vi "BX.Init__LCR.vi"(3 "Container State":T10, 4 "Previous State":variant, 5 "Previous Version":T9) -> (2 "Current State":T1={"Orientation"=0, "ActivePicture"={"image type"=0, "image depth"=0, "image"=[], "mask"=[], "colors"=[], "Rectangle"={"left"=0, "top"=0, "right"=0, "bottom"=0}}, "Pictures"={"Normal"={"image type"=0, "image depth"=0, "image"=[], "mask"=[], "colors"=[], "Rectangle"={"left"=0, "top"=0, "right"=0, "bottom"=0}}, "Hilite"={"image type"=0, "image depth"=0, "image"=[], "mask"=[], "colors"=[], "Rectangle"={"left"=0, "top"=0, "right"=0, "bottom"=0}}}, "Text"={"String"="", "Font"={"Font Name:"="", "Size"=0, "Strikeout?"=FALSE, "Italic?"=FALSE, "Underline?"=FALSE, "Outline?"=FALSE, "Shadow?"=FALSE, "Bold?"=FALSE}, "TextColor"=0}, "RunTimeSettings"={"Highlight"=FALSE, "ShowButton"=TRUE, "Behaviour"=enum."Switch when pressed", "React if disabled"=FALSE, "Nudge Button"=TRUE, "ShowButton on Hover"=FALSE, "Button Type"=enum."System"}, "Messages"=[], "Status"=0, "XControl Label"="", "Boolean Value"=FALSE} {"Status" format="%.0x"})   [LabVIEW 2011, in "BooleanXControl__LCR.xctl"]
doc: "Loads data from the owning VI into the XControl"
uses:
  BooleanXControl__LCR.xctl
  BX.State__LCR.ctl
  Controls/BX.Orientation__LCR.ctl
  <vilib>/picture/picture.llb/imagedata.ctl
  Controls/BX.RTSettings__LCR.ctl
  Controls/BX.Behaviour__LCR.ctl
  Controls/BX.ButtonType__LCR.ctl
  Controls/BX.Message__LCR.ctl
  Controls/BX.Commands__LCR.ctl
  <vilib>/_xctls/Container State.ctl
  <vilib>/_xctls/Version.ctl
  <vilib>/_xctls/XControlSupport.lvlib
panel:
  in  "Default Indicator State":T1={"Orientation"=0, "ActivePicture"={"image type"=0, "image depth"=0, "image"=[], "mask"=[], "colors"=[], "Rectangle"={"left"=0, "top"=0, "right"=0, "bottom"=0}}, "Pictures"={"Normal"={"image type"=0, "image depth"=0, "image"=[], "mask"=[], "colors"=[], "Rectangle"={"left"=0, "top"=0, "right"=0, "bottom"=0}}, "Hilite"={"image type"=0, "image depth"=0, "image"=[], "mask"=[], "colors"=[], "Rectangle"={"left"=0, "top"=0, "right"=0, "bottom"=0}}}, "Text"={"String"="", "Font"={"Font Name:"="", "Size"=10, "Strikeout?"=FALSE, "Italic?"=FALSE, "Underline?"=FALSE, "Outline?"=FALSE, "Shadow?"=FALSE, "Bold?"=FALSE}, "TextColor"=0}, "RunTimeSettings"={"Highlight"=TRUE, "ShowButton"=TRUE, "Behaviour"=enum."Switch when pressed", "React if disabled"=FALSE, "Nudge Button"=TRUE, "ShowButton on Hover"=FALSE, "Button Type"=enum."System"}, "Messages"=[], "Status"=0, "XControl Label"="", "Boolean Value"=FALSE} {"Status" format="%.0x"}
  in  "Default Control State":T1={"Orientation"=0, "ActivePicture"={"image type"=0, "image depth"=0, "image"=[], "mask"=[], "colors"=[], "Rectangle"={"left"=0, "top"=0, "right"=0, "bottom"=0}}, "Pictures"={"Normal"={"image type"=0, "image depth"=0, "image"=[], "mask"=[], "colors"=[], "Rectangle"={"left"=0, "top"=0, "right"=0, "bottom"=0}}, "Hilite"={"image type"=0, "image depth"=0, "image"=[], "mask"=[], "colors"=[], "Rectangle"={"left"=0, "top"=0, "right"=0, "bottom"=0}}}, "Text"={"String"="", "Font"={"Font Name:"="", "Size"=10, "Strikeout?"=FALSE, "Italic?"=FALSE, "Underline?"=FALSE, "Outline?"=FALSE, "Shadow?"=FALSE, "Bold?"=FALSE}, "TextColor"=0}, "RunTimeSettings"={"Highlight"=TRUE, "ShowButton"=TRUE, "Behaviour"=enum."Switch when pressed", "React if disabled"=FALSE, "Nudge Button"=TRUE, "ShowButton on Hover"=FALSE, "Button Type"=enum."System"}, "Messages"=[], "Status"=0, "XControl Label"="", "Boolean Value"=FALSE} {"Status" format="%.0x"}
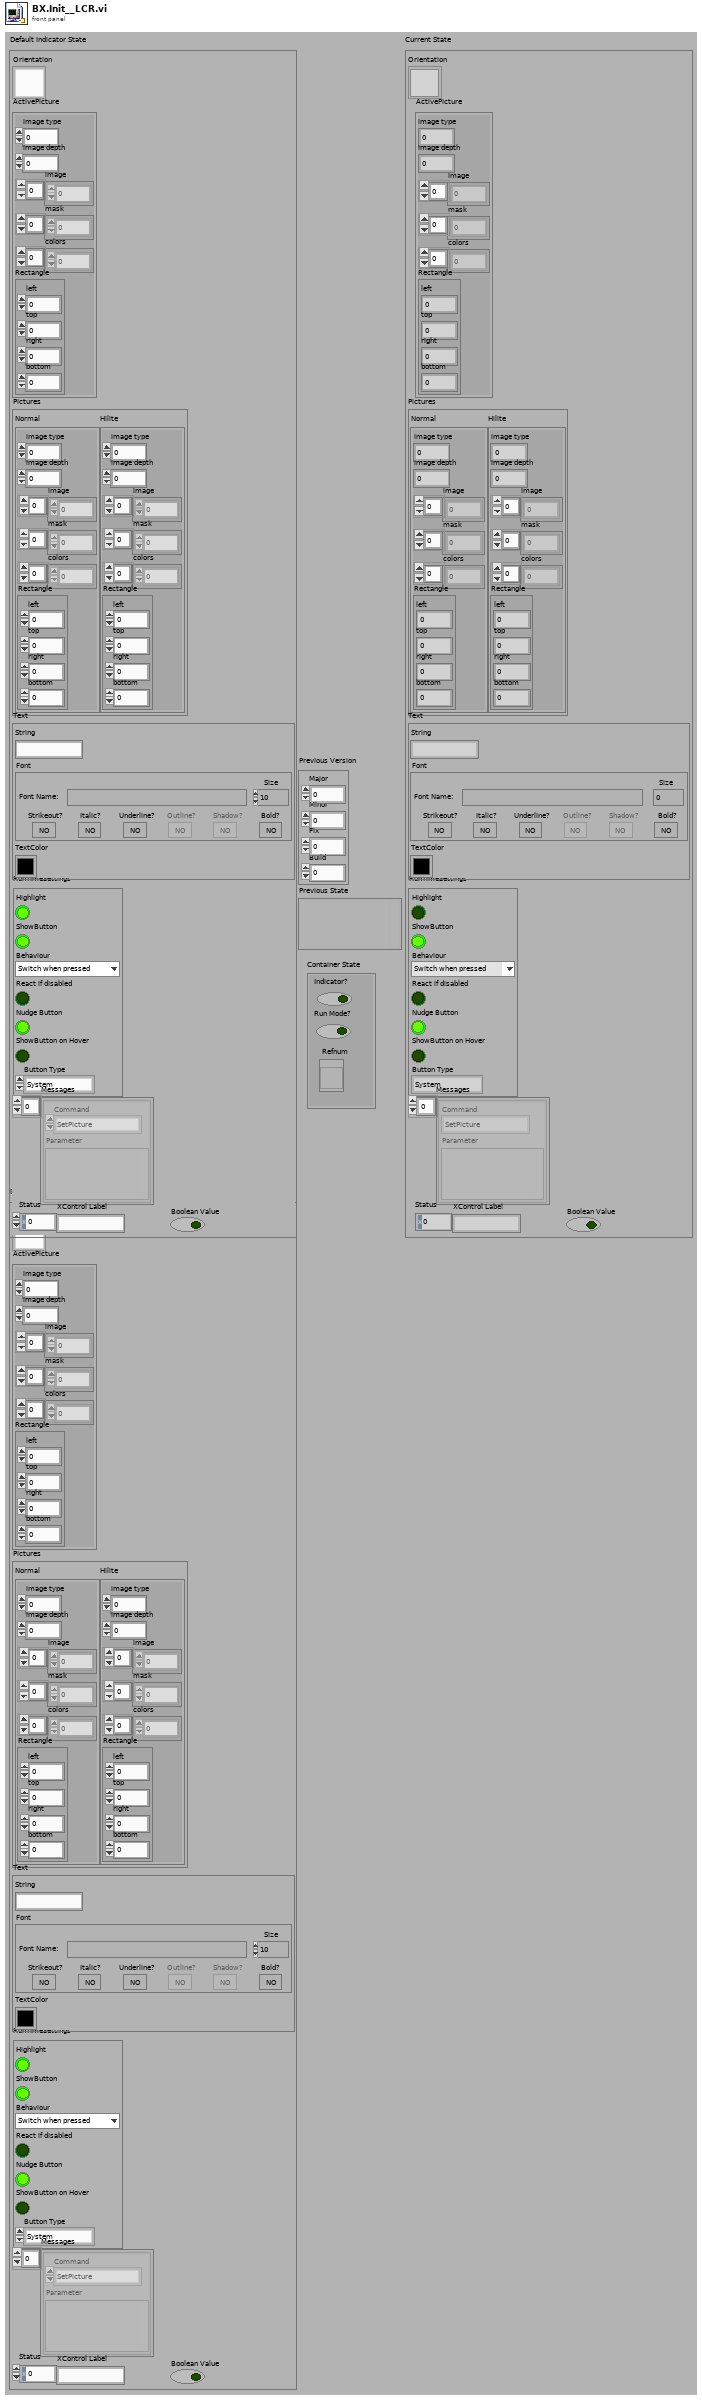
[diagram p1: front panel]
types:
  T1 = typedef "BooleanXControl__LCR.xctl/BX.State__LCR.ctl" = cluster{"Orientation":T2, "ActivePicture":T3, "Pictures":cluster{"Normal":T3, "Hilite":T3}, "Text":cluster{"String":string, "Font":cluster{"Font Name:":string, "Size":i16, "Strikeout?":bool, "Italic?":bool, "Underline?":bool, "Outline?":bool, "Shadow?":bool, "Bold?":bool}, "TextColor":u32}, "RunTimeSettings":T4, "Messages":T7[], "Status":u16, "XControl Label":string, "Boolean Value":bool}
  T2 = typedef "BooleanXControl__LCR.xctl/BX.Orientation__LCR.ctl" = u8
  T3 = typedef "imagedata.ctl" = cluster{"image type":i32, "image depth":i32, "image":u8[], "mask":u8[], "colors":u32[], "Rectangle":cluster{"left":i16, "top":i16, "right":i16, "bottom":i16}}
  T4 = typedef "BooleanXControl__LCR.xctl/BX.RTSettings__LCR.ctl" = cluster{"Highlight":bool, "ShowButton":bool, "Behaviour":T5, "React if disabled":bool, "Nudge Button":bool, "ShowButton on Hover":bool, "Button Type":T6}
  T5 = typedef "BooleanXControl__LCR.xctl/BX.Behaviour__LCR.ctl" = enum16{"Switch when pressed", "Switch when released", "Switch until released"}
  T6 = typedef "BooleanXControl__LCR.xctl/BX.ButtonType__LCR.ctl" = enum16{"System", "Modern", "Classic", "Decoration"}
  T7 = typedef "BooleanXControl__LCR.xctl/BX.Message__LCR.ctl" = cluster{"Command":T8, "Parameter":variant}
  T8 = typedef "BooleanXControl__LCR.xctl/BX.Commands__LCR.ctl" = enum16{"None", "SetPicture", "SetFont", "SetText", "SetOrientation", "Redraw", "SetTextColor", "SetRTSettings", "MultipleUpdate", "RT.Button", "RT.Hilite", "RT.Behaviour", "RT.Disabled", "ShowGUI", "RT.Nudge", "RT.Hover", "RT.ButtonType"}
  T9 = typedef "XControlSupport.lvlib/Version.ctl" = cluster{"Major":u16, "Minor":u16, "Fix":u16, "Build":u16}
  T10 = typedef "XControlSupport.lvlib/Container State.ctl" = cluster{"Indicator?":bool, "Run Mode?":bool, " Refnum":refnum<vi>}
  T11 = cluster{"Orientation":u8, "ActivePicture":cluster{"image type":i32, "image depth":i32, "image":u8[], "mask":u8[], "colors":u32[], "Rectangle":cluster{"left":i16, "top":i16, "right":i16, "bottom":i16}}, "Pictures":cluster{"Normal":cluster{"image type":i32, "image depth":i32, "image":u8[], "mask":u8[], "colors":u32[], "Rectangle":cluster{"left":i16, "top":i16, "right":i16, "bottom":i16}}, "Hilite":cluster{"image type":i32, "image depth":i32, "image":u8[], "mask":u8[], "colors":u32[], "Rectangle":cluster{"left":i16, "top":i16, "right":i16, "bottom":i16}}}, "Text":cluster{"String":string, "Font":cluster{"Font Name:":string, "Size":i16, "Strikeout?":bool, "Italic?":bool, "Underline?":bool, "Outline?":bool, "Shadow?":bool, "Bold?":bool}, "TextColor":u32}, "RunTimeSettings":cluster{"Highlight":bool, "ShowButton":bool, "Behaviour":T5, "React if disabled":bool}, "Messages":cluster{"Command":enum16{"None", "SetPicture", "SetFont", "SetText", "SetOrientation", "Redraw", "SetTextColor", "SetRTSettings", "MultipleUpdate", "RT.Button", "RT.Hilite", "RT.Behaviour", "RT.Disabled", "ShowGUI"}, "Parameter":variant}[], "Status":u16, "XControl Label":string}
  T12 = cluster{"Orientation":u8, "ActivePicture":cluster{"image type":i32, "image depth":i32, "image":u8[], "mask":u8[], "colors":u32[], "Rectangle":cluster{"left":i16, "top":i16, "right":i16, "bottom":i16}}, "Pictures":cluster{"Normal":cluster{"image type":i32, "image depth":i32, "image":u8[], "mask":u8[], "colors":u32[], "Rectangle":cluster{"left":i16, "top":i16, "right":i16, "bottom":i16}}, "Hilite":cluster{"image type":i32, "image depth":i32, "image":u8[], "mask":u8[], "colors":u32[], "Rectangle":cluster{"left":i16, "top":i16, "right":i16, "bottom":i16}}}, "Text":cluster{"String":string, "Font":cluster{"Font Name:":string, "Size":i16, "Strikeout?":bool, "Italic?":bool, "Underline?":bool, "Outline?":bool, "Shadow?":bool, "Bold?":bool}, "TextColor":u32}, "RunTimeSettings":cluster{"Highlight":bool, "ShowButton":bool, "Behaviour":enum16{"Switch when pressed", "Switch when released", "Switch until released"}, "React if disabled":bool}, "Messages":cluster{"Command":T8, "Parameter":variant}, "Status":u16, "XControl Label":string, "Events (DO NOT DESTROY)":cluster{"user event":refnum<user-event>, "Event Registration Refnum":refnum<event-registration>}}
  T13 = cluster{"Orientation":u8, "ActivePicture":cluster{"image type":i32, "image depth":i32, "image":u8[], "mask":u8[], "colors":u32[], "Rectangle":cluster{"left":i16, "top":i16, "right":i16, "bottom":i16}}, "Pictures":cluster{"Normal":cluster{"image type":i32, "image depth":i32, "image":u8[], "mask":u8[], "colors":u32[], "Rectangle":cluster{"left":i16, "top":i16, "right":i16, "bottom":i16}}, "Hilite":cluster{"image type":i32, "image depth":i32, "image":u8[], "mask":u8[], "colors":u32[], "Rectangle":cluster{"left":i16, "top":i16, "right":i16, "bottom":i16}}}, "Text":cluster{"String":string, "Font":cluster{"Font Name:":string, "Size":i16, "Strikeout?":bool, "Italic?":bool, "Underline?":bool, "Outline?":bool, "Shadow?":bool, "Bold?":bool}, "TextColor":u32}, "RunTimeSettings":cluster{"Highlight":bool, "ShowButton":bool, "Behaviour":enum16{"Switch when pressed", "Switch when released", "Switch until released"}, "React if disabled":bool}, "Messages":cluster{"Command":enum16{"None", "SetPicture", "SetFont", "SetText", "SetOrientation", "Redraw", "SetTextColor", "SetRTSettings", "MultipleUpdate", "RT.Button", "RT.Hilite", "RT.Behaviour", "RT.Disabled", "ShowGUI"}, "Parameter":variant}, "Status":u16}
  T14 = cluster{"Orientation":u8, "ActivePicture":cluster{"image type":i32, "image depth":i32, "image":u8[], "mask":u8[], "colors":u32[], "Rectangle":cluster{"left":i16, "top":i16, "right":i16, "bottom":i16}}, "Pictures":cluster{"Normal":cluster{"image type":i32, "image depth":i32, "image":u8[], "mask":u8[], "colors":u32[], "Rectangle":cluster{"left":i16, "top":i16, "right":i16, "bottom":i16}}, "Hilite":cluster{"image type":i32, "image depth":i32, "image":u8[], "mask":u8[], "colors":u32[], "Rectangle":cluster{"left":i16, "top":i16, "right":i16, "bottom":i16}}}, "Text":cluster{"String":string, "Font":cluster{"Font Name:":string, "Size":i16, "Strikeout?":bool, "Italic?":bool, "Underline?":bool, "Outline?":bool, "Shadow?":bool, "Bold?":bool}, "TextColor":u32}, "RunTimeSettings":cluster{"Highlight":bool, "ShowButton":bool, "Behaviour":enum16{"Switch when pressed", "Switch when released", "Switch until released"}, "React if disabled":bool}, "Messages":cluster{"Command":enum16{"None", "SetPicture", "SetFont", "SetText", "SetOrientation", "Redraw", "SetTextColor", "SetRTSettings", "MultipleUpdate", "RT.Button", "RT.Hilite", "RT.Behaviour", "RT.Disabled", "ShowGUI"}, "Parameter":variant}, "Spacing":u8}
  T15 = cluster{"image type":i32, "image depth":i32, "image":u8[], "mask":u8[], "colors":u32[], "Rectangle":cluster{"left":i16, "top":i16, "right":i16, "bottom":i16}}
  T16 = cluster{"Normal":cluster{"image type":i32, "image depth":i32, "image":u8[], "mask":u8[], "colors":u32[], "Rectangle":cluster{"left":i16, "top":i16, "right":i16, "bottom":i16}}, "Hilite":cluster{"image type":i32, "image depth":i32, "image":u8[], "mask":u8[], "colors":u32[], "Rectangle":cluster{"left":i16, "top":i16, "right":i16, "bottom":i16}}}
  T17 = cluster{"String":string, "Font":cluster{"Font Name:":string, "Size":i16, "Strikeout?":bool, "Italic?":bool, "Underline?":bool, "Outline?":bool, "Shadow?":bool, "Bold?":bool}, "TextColor":u32}
  T18 = cluster{"Highlight":bool, "ShowButton":bool, "Behaviour":enum16{"Switch when pressed", "Switch when released", "Switch until released"}, "React if disabled":bool}
  T19 = cluster{"Command":enum16{"None", "SetPicture", "SetFont", "SetText", "SetOrientation", "Redraw", "SetTextColor", "SetRTSettings", "MultipleUpdate", "RT.Button", "RT.Hilite", "RT.Behaviour", "RT.Disabled", "ShowGUI"}, "Parameter":variant}
  T20 = enum16{"Switch when pressed", "Switch when released", "Switch until released"}
  T21 = cluster{"Command":enum16{"None", "SetPicture", "SetFont", "SetText", "SetOrientation", "Redraw", "SetTextColor", "SetRTSettings", "MultipleUpdate", "RT.Button", "RT.Hilite", "RT.Behaviour", "RT.Disabled", "ShowGUI"}, "Parameter":variant}[]
  T22 = cluster{"Highlight":bool, "ShowButton":bool, "Behaviour":enum16{"Switch when pressed", "Switch when released", "Switch until released"}, "React if disabled":bool, bool, bool, "Button Type":T6}
  T23 = cluster{"Highlight":bool, "ShowButton":bool, "Behaviour":T5, "React if disabled":bool}
  T24 = cluster{"Highlight":bool, "ShowButton":bool, "Behaviour":T5, "React if disabled":bool, bool, bool, "Button Type":T6}
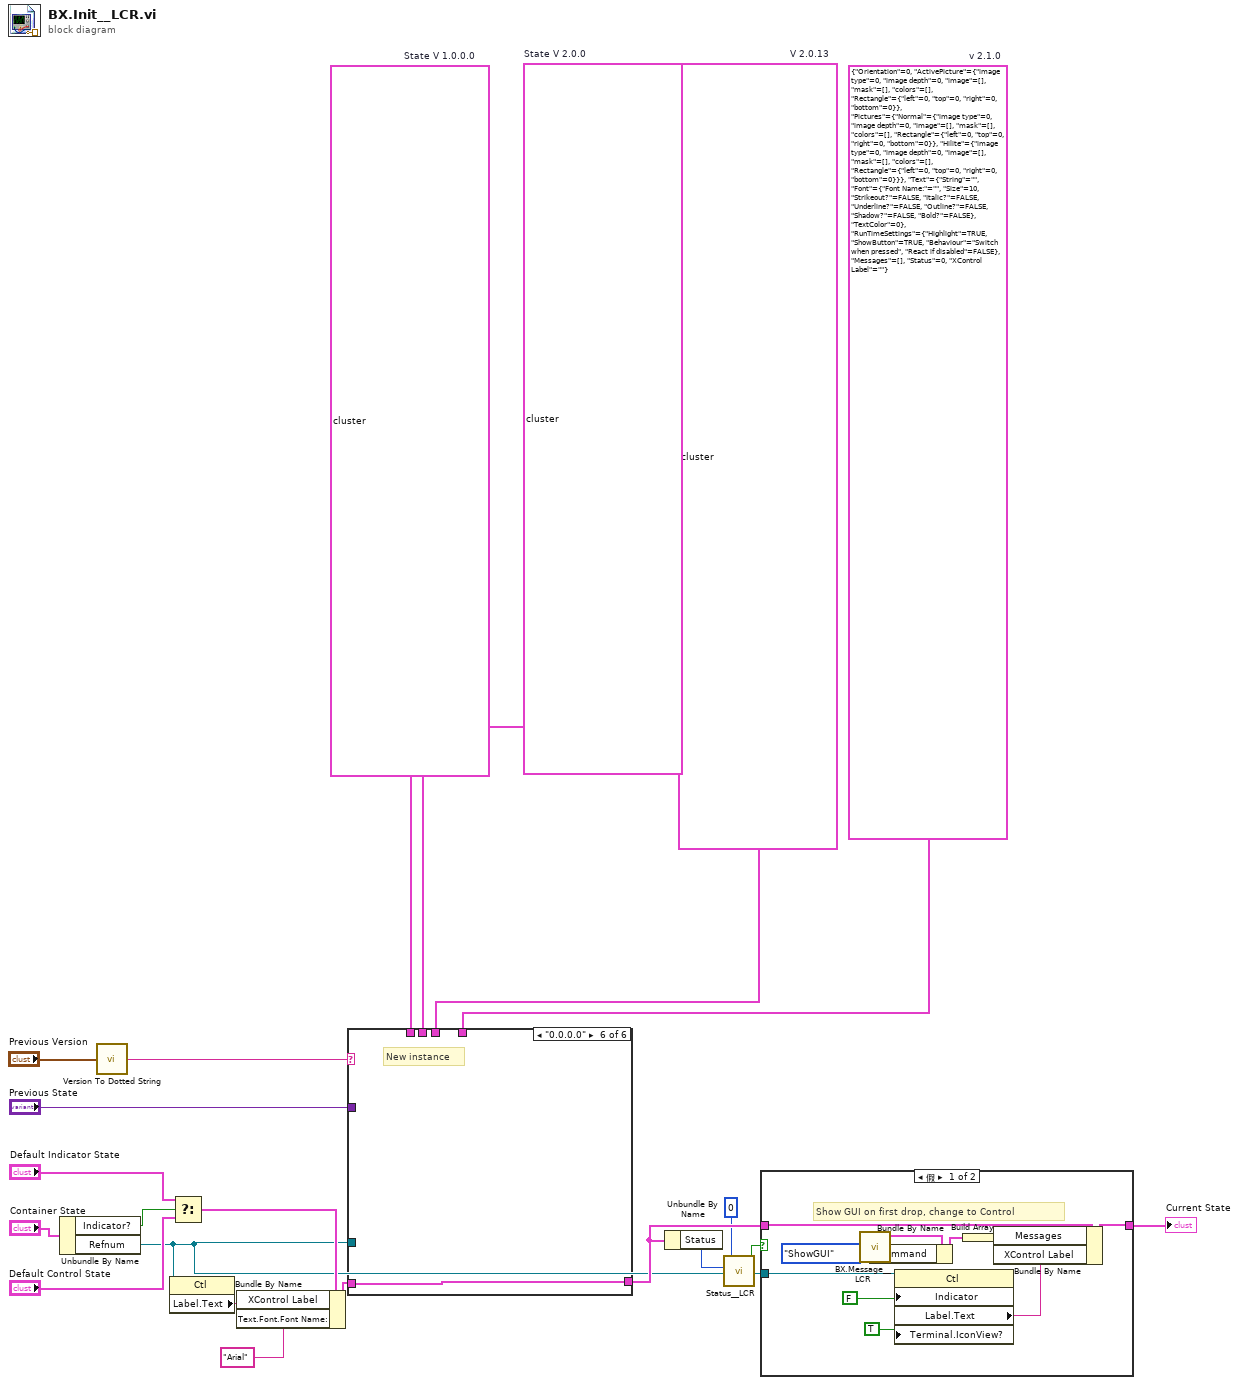
[diagram p0: block diagram]
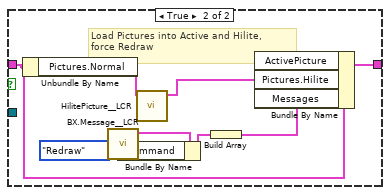
[diagram p2: hidden frame]
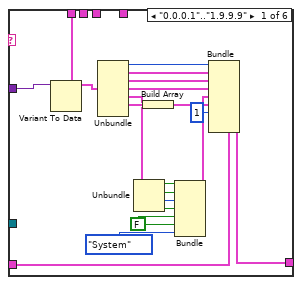
[diagram p3: hidden frame]
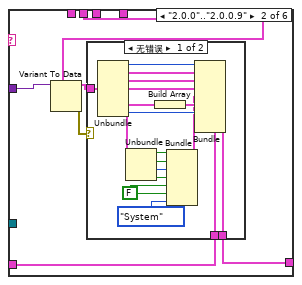
[diagram p4: hidden frame]
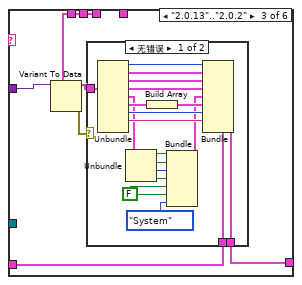
[diagram p6: hidden frame]
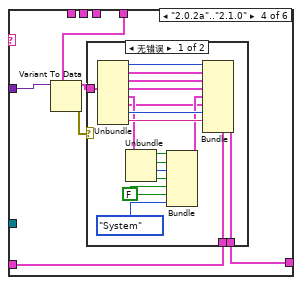
[diagram p8: hidden frame]
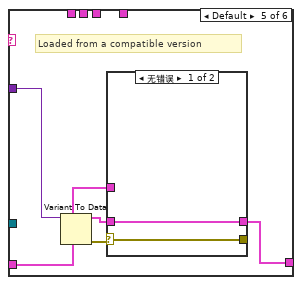
[diagram p10: hidden frame]
diagram:
  w6 = T11 {"Orientation"=0, "ActivePicture"={"image type"=0, "image depth"=0, "image"=[], "mask"=[], "colors"=[], "Rectangle"={"left"=0, "top"=0, "right"=0, "bottom"=0}}, "Pictures"={"Normal"={"image type"=0, "image depth"=0, "image"=[], "mask"=[], "colors"=[], "Rectangle"={"left"=0, "top"=0, "right"=0, "bottom"=0}}, "Hilite"={"image type"=0, "image depth"=0, "image"=[], "mask"=[], "colors"=[], "Rectangle"={"left"=0, "top"=0, "right"=0, "bottom"=0}}}, "Text"={"String"="", "Font"={"Font Name:"="", "Size"=10, "Strikeout?"=FALSE, "Italic?"=FALSE, "Underline?"=FALSE, "Outline?"=FALSE, "Shadow?"=FALSE, "Bold?"=FALSE}, "TextColor"=0}, "RunTimeSettings"={"Highlight"=TRUE, "ShowButton"=TRUE, "Behaviour"=enum."Switch when pressed", "React if disabled"=FALSE}, "Messages"=[], "Status"=0, "XControl Label"=""}  # v 2.1.0
  w9 = T12 {"Orientation"=0, "ActivePicture"={"image type"=0, "image depth"=0, "image"=[], "mask"=[], "colors"=[], "Rectangle"={"left"=0, "top"=0, "right"=0, "bottom"=0}}, "Pictures"={"Normal"={"image type"=0, "image depth"=0, "image"=[], "mask"=[], "colors"=[], "Rectangle"={"left"=0, "top"=0, "right"=0, "bottom"=0}}, "Hilite"={"image type"=0, "image depth"=0, "image"=[], "mask"=[], "colors"=[], "Rectangle"={"left"=0, "top"=0, "right"=0, "bottom"=0}}}, "Text"={"String"="", "Font"={"Font Name:"="", "Size"=10, "Strikeout?"=FALSE, "Italic?"=FALSE, "Underline?"=FALSE, "Outline?"=FALSE, "Shadow?"=FALSE, "Bold?"=FALSE}, "TextColor"=0}, "RunTimeSettings"={"Highlight"=TRUE, "ShowButton"=TRUE, "Behaviour"=enum."Switch when pressed", "React if disabled"=FALSE}, "Messages"={"Command"=enum."SetPicture", "Parameter"=variant}, "Status"=0, "XControl Label"="", "Events (DO NOT DESTROY)"={"user event"=refnum, "Event Registration Refnum"=refnum}}  # V 2.0.13
  w12 = T13 {"Orientation"=0, "ActivePicture"={"image type"=0, "image depth"=0, "image"=[], "mask"=[], "colors"=[], "Rectangle"={"left"=0, "top"=0, "right"=0, "bottom"=0}}, "Pictures"={"Normal"={"image type"=0, "image depth"=0, "image"=[], "mask"=[], "colors"=[], "Rectangle"={"left"=0, "top"=0, "right"=0, "bottom"=0}}, "Hilite"={"image type"=0, "image depth"=0, "image"=[], "mask"=[], "colors"=[], "Rectangle"={"left"=0, "top"=0, "right"=0, "bottom"=0}}}, "Text"={"String"="", "Font"={"Font Name:"="", "Size"=0, "Strikeout?"=FALSE, "Italic?"=FALSE, "Underline?"=FALSE, "Outline?"=FALSE, "Shadow?"=FALSE, "Bold?"=FALSE}, "TextColor"=0}, "RunTimeSettings"={"Highlight"=FALSE, "ShowButton"=TRUE, "Behaviour"=enum."Switch when pressed", "React if disabled"=FALSE}, "Messages"={"Command"=enum."SetPicture", "Parameter"=variant}, "Status"=0}  # State V 2.0.0
  w7 = T14 {"Orientation"=0, "ActivePicture"={"image type"=0, "image depth"=0, "image"=[], "mask"=[], "colors"=[], "Rectangle"={"left"=0, "top"=0, "right"=0, "bottom"=0}}, "Pictures"={"Normal"={"image type"=0, "image depth"=0, "image"=[], "mask"=[], "colors"=[], "Rectangle"={"left"=0, "top"=0, "right"=0, "bottom"=0}}, "Hilite"={"image type"=0, "image depth"=0, "image"=[], "mask"=[], "colors"=[], "Rectangle"={"left"=0, "top"=0, "right"=0, "bottom"=0}}}, "Text"={"String"="", "Font"={"Font Name:"="", "Size"=0, "Strikeout?"=FALSE, "Italic?"=FALSE, "Underline?"=FALSE, "Outline?"=FALSE, "Shadow?"=FALSE, "Bold?"=FALSE}, "TextColor"=0}, "RunTimeSettings"={"Highlight"=FALSE, "ShowButton"=TRUE, "Behaviour"=enum."Switch when pressed", "React if disabled"=FALSE}, "Messages"={"Command"=enum."SetPicture", "Parameter"=variant}, "Spacing"=0}  # State V 1.0.0.0
  n1 = Unbundle By Name("Container State") -> ("Indicator?"=w17:bool, "Refnum"=w11:refnum<vi>)
  n2 = call <vilib>:"Version To Dotted String.vi"("Version"="Previous Version") -> ("String Version"=w14:string)
  n3 = property class="Ctl"(reference=w11) -> ("Label.Text"=w10:string)  [unwired: 1 in, 2 out]
  n4 = Select(t="Default Indicator State", s=w17, f="Default Control State") -> (s? t:f=w16:T1)
  n5 = Bundle By Name(cluster=w16, "XControl Label"=w10, "Text.Font.Font Name:"="Arial") -> (w5:T1)
  n6 = case shown="\"0.0.0.0\"" w14 {
    tunnel: "Previous State" -> [w41 w47 w72 w98 w122 _]
    tunnel: [w37 w42 w68 w94 w118 w127] -> w13
    tunnel: w5 -> [w38 w45 w70 w96 w119 w127]
    tunnel: w7 -> [w40 _ _ _ _ _]
    tunnel: w12 -> [_ w44 _ _ _ _]
    tunnel: w11 -> [_ _ _ _ _ _]
    tunnel: w9 -> [_ _ w67 _ _ _]
    tunnel: w6 -> [_ _ _ w93 _ _]
    frame "0.0.0.1".."1.9.9.9" {
      w25 = FALSE
      n7 = Variant To Data(type=w40, Variant=w41) -> (data=w39:T14)  [unwired: 1 in, 1 out]
      n8 = Unbundle(w39) -> ("Orientation"=w36:u8, "ActivePicture"=w35:T15, "Pictures"=w34:T16, "Text"=w33:T17, "RunTimeSettings"=w24:T18, "Messages"=w32:T19)  [unwired: 1 out]
      n9 = Unbundle(w24) -> ("Highlight"=w29:bool, "ShowButton"=w28:bool, "Behaviour"=w27:T20, "React if disabled"=w26:bool)
      n10 = Build Array(w32) -> (w30:T21)
      n11 = Bundle("Highlight"=w29, "ShowButton"=w28, "Behaviour"=w27, "React if disabled"=w26, w25, w25, "Button Type"=BX.ButtonType__LCR."System") -> (w23:T22)  [unwired: 1 in]
      n12 = Bundle(cluster=w38, "Orientation"=w36, "ActivePicture"=w35, "Pictures"=w34, "Text"=w33, "RunTimeSettings"=w23, "Messages"=w30, "Status"=u16 1) -> (w37:T1)  [unwired: 2 in]
    }
    frame "2.0.0".."2.0.0.9" {
      n13 = Variant To Data(type=w44, Variant=w47) -> (data=w46:T13, error out=w43:errorcluster)  [unwired: 1 in]
      n14 = case shown="无错误" w43 {
        tunnel: w46 -> [w65 _]
        tunnel: w45 -> [w64 w66]
        tunnel: [w63 w66] -> w42
        frame No Error {
          w51 = FALSE
          n15 = Unbundle(w65) -> ("Orientation"=w62:u8, "ActivePicture"=w61:T15, "Pictures"=w60:T16, "Text"=w59:T17, "RunTimeSettings"=w50:T18, "Messages"=w58:T19, "Status"=w57:u16)
          n16 = Unbundle(w50) -> ("Highlight"=w55:bool, "ShowButton"=w54:bool, "Behaviour"=w53:T20, "React if disabled"=w52:bool)
          n17 = Build Array(w58) -> (w56:T21)
          n18 = Bundle("Highlight"=w55, "ShowButton"=w54, "Behaviour"=w53, "React if disabled"=w52, w51, w51, "Button Type"=BX.ButtonType__LCR."System") -> (w49:T22)  [unwired: 1 in]
          n19 = Bundle(cluster=w64, "Orientation"=w62, "ActivePicture"=w61, "Pictures"=w60, "Text"=w59, "RunTimeSettings"=w49, "Messages"=w56, "Status"=w57) -> (w63:T1)  [unwired: 2 in]
        }
        frame Error {
        }
      }
    }
    frame "2.0.13".."2.0.2" {
      n20 = Variant To Data(type=w67, Variant=w72) -> (data=w71:T12, error out=w69:errorcluster)  [unwired: 1 in]
      n21 = case shown="无错误" w69 {
        tunnel: w71 -> [w91 _]
        tunnel: w70 -> [w90 w92]
        tunnel: [w89 w92] -> w68
        frame No Error {
          w74 = FALSE
          n22 = Unbundle(w91) -> ("Orientation"=w88:u8, "ActivePicture"=w87:T15, "Pictures"=w86:T16, "Text"=w85:T17, "RunTimeSettings"=w80:T18, "Messages"=w84:cluster{"Command":T8, "Parameter":variant}, "Status"=w83:u16, "XControl Label"=w81:string)  [unwired: 1 out]
          n23 = Unbundle(w80) -> ("Highlight"=w79:bool, "ShowButton"=w77:bool, "Behaviour"=w76:T20, "React if disabled"=w75:bool)
          n24 = Build Array(w84) -> (w82:cluster{"Command":T8, "Parameter":variant}[])
          n25 = Bundle("Highlight"=w79, "ShowButton"=w77, "Behaviour"=w76, "React if disabled"=w75, w74, w74, "Button Type"=BX.ButtonType__LCR."System") -> (w78:T22)  [unwired: 1 in]
          n26 = Bundle(cluster=w90, "Orientation"=w88, "ActivePicture"=w87, "Pictures"=w86, "Text"=w85, "RunTimeSettings"=w78, "Messages"=w82, "Status"=w83, "XControl Label"=w81) -> (w89:T1)  [unwired: 1 in]
        }
        frame Error {
        }
      }
    }
    frame "2.0.2a".."2.1.0" {
      n27 = Variant To Data(type=w93, Variant=w98) -> (data=w97:T11, error out=w95:errorcluster)  [unwired: 1 in]
      n28 = case shown="无错误" w95 {
        tunnel: w97 -> [w116 _]
        tunnel: w96 -> [w115 w117]
        tunnel: [w114 w117] -> w94
        frame No Error {
          w101 = FALSE
          n29 = Unbundle(w116) -> ("Orientation"=w113:u8, "ActivePicture"=w112:T15, "Pictures"=w111:T16, "Text"=w110:T17, "RunTimeSettings"=w107:T23, "Messages"=w100:T21, "Status"=w109:u16, "XControl Label"=w108:string)
          n30 = Unbundle(w107) -> ("Highlight"=w106:bool, "ShowButton"=w104:bool, "Behaviour"=w103:T5, "React if disabled"=w102:bool)
          n31 = Bundle("Highlight"=w106, "ShowButton"=w104, "Behaviour"=w103, "React if disabled"=w102, w101, w101, "Button Type"=BX.ButtonType__LCR."System") -> (w105:T24)  [unwired: 1 in]
          n32 = Bundle(cluster=w115, "Orientation"=w113, "ActivePicture"=w112, "Pictures"=w111, "Text"=w110, "RunTimeSettings"=w105, "Messages"=w100, "Status"=w109, "XControl Label"=w108) -> (w114:T1)  [unwired: 1 in]
        }
        frame Error {
        }
      }
    }
    frame Default {
      # "Loaded from a compatible version"
      n33 = Variant To Data(type=w119, Variant=w122) -> (data=w120:T1, error out=w121:errorcluster)  [unwired: 1 in]
      n34 = case shown="无错误" w121 {
        selector: w121 -> [w124 w125]
        tunnel: w120 -> [w123 _]
        tunnel: [w123 w126] -> w118
        tunnel: w119 -> [_ w126]
        tunnel: [w124 w125] -> _
        frame No Error {
        }
        frame Error {
          # "Or not so compatible"
        }
      }
    }
    frame "0.0.0.0" {
      # "New instance"
    }
  }
  n35 = Unbundle By Name(w13) -> ("Status"=w4:u16)
  n36 = call "Status__LCR.vi"("Status In"=w4, "Bit"=u16 0) -> ("Bit Value Out"=w3:bool)  [unwired: 8 in, 1 out]
  n37 = case shown="假" w3 {
    tunnel: w13 -> [w135 w143]
    tunnel: [w134 w142] -> w8
    tunnel: w11 -> [w137 _]
    frame False {
      # "Show GUI on first drop, change to Control"
      n38 = call "BX.Message__LCR.vi"() -> ("Messages"=w131:T7)  [unwired: 11 in]
      n39 = Bundle By Name(cluster=w131, "Command"=BX.Commands__LCR."ShowGUI" ("Messages.Command")) -> (w130:T7)
      n40 = property class="Ctl"(reference=w137, "Indicator"=FALSE, "Terminal.IconView?"=TRUE ("Terminal.Icon View?")) -> ("Label.Text"=w133:string)  [unwired: 1 in, 2 out]
      n41 = Build Array(w130) -> (w129:T7[])
      n42 = Bundle By Name(cluster=w135, "Messages"=w129, "XControl Label"=w133) -> (w134:T1)
    }
    frame True {
      # "Load Pictures into Active and Hilite,\nforce Redraw"
      n43 = Unbundle By Name(w143) -> ("Pictures.Normal"=w145:T3)
      n44 = call "BX.Message__LCR.vi"() -> ("Messages"=w140:T7)  [unwired: 11 in]
      n45 = Bundle By Name(cluster=w140, "Command"=BX.Commands__LCR."Redraw" ("Messages.Command")) -> (w139:T7)
      n46 = call "HilitePicture__LCR.vi"("image data"=w145) -> ("Hilited Picture"=w144:T3)  [unwired: 9 in, 1 out]
      n47 = Build Array(w139) -> (w138:T7[])
      n48 = Bundle By Name(cluster=w143, "ActivePicture"=w145, "Pictures.Hilite"=w144, "Messages"=w138) -> (w142:T1)
    }
  }
  "Current State" <- w8
